vi "unmarshalling.vi"(7 "Type":variant, 8 "error in (no error)":errorcluster, 10 "String":string, 11 "Serializer in":refnum<class "Serializer.openg-ini.lvclass">) -> (0 "error out":errorcluster, 2 "Variant":variant, 3 "Serializer":refnum<class "Serializer.openg-ini.lvclass">)   [LabVIEW 2019, in "OpenSerializer.OpenG-ini.lvlib" / "Serializer.openg-ini.lvclass"]
uses:
  Serializer.openg-ini.lvclass
  Serializer.openg-ini.lvclass/Serializer.openg-ini.ctl
  <vilib>/Utility/config.llb/NI_LVConfig.lvlib
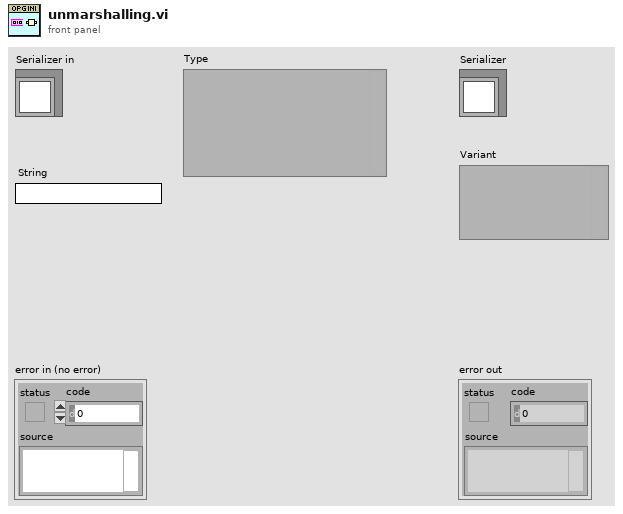
[diagram p1: front panel]
types:
  T1 = enum16{"open", "replace", "create", "open or create", "replace or create", "replace or create with confirmation"}
  T2 = typedef "NI_LVConfig.lvlib/Config Data RefNum.ctl" = refnum<k1>
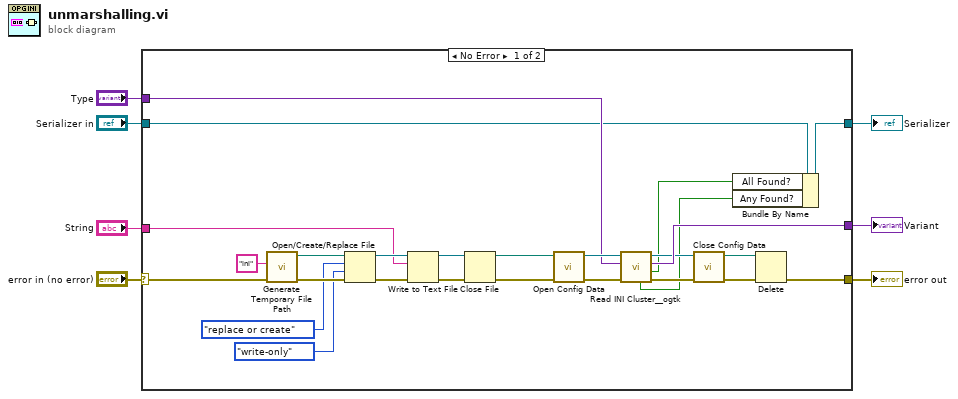
[diagram p0: block diagram]
diagram:
  n1 = case shown="No Error" "error in (no error)" {
    selector: "error in (no error)" -> [w32 w34]
    tunnel: "Serializer in" -> [w11 w35]
    tunnel: "String" -> [w25 _]
    tunnel: [w12 w35] -> w5
    tunnel: [w9 w34] -> w4
    tunnel: [w16 _] -> w3
    tunnel: "Type" -> [w17 _]
    frame No Error {
      n2 = call <vilib>:"Generate Temporary File Path.vi"("error in (no error)"=w32, "Temporary File Extension (tmp)"="ini") -> ("error out"=w30:errorcluster, "Unique Temporary File Path"=w31:path)  [unwired: 8 in]
      n3 = Open/Create/Replace File(file path (use dialog)=w31, error in=w30, operation (0:open)=T1."replace or create", access (0:read/write)=enum16{"read/write", "read-only", "write-only"}."write-only") -> (refnum out=w27:refnum<file>, error out=w26:errorcluster)  [unwired: 2 in, 1 out]
      n4 = Write to Text File(file (use dialog)=w27, text=w25, error in=w26) -> (refnum out=w23:refnum<file>, error out=w24:errorcluster)  [unwired: 1 in, 1 out]
      n5 = Close File(refnum=w23, error in=w24) -> (path=w21:path, error out=w22:errorcluster)
      n6 = call <vilib>:"Open Config Data.vi"("error in (no error)"=w22, "configuration file path"=w21) -> ("error out"=w20:errorcluster, "refnum"=w18:T2)  [unwired: 7 in, 1 out]
      n7 = call <userlib>:"Read INI Cluster__ogtk.vi"("error in (no error)"=w20, "INI Fomatted Cluster Type"=w17, "refnum"=w18) -> ("error out"=w19:errorcluster, "all found?"=w14:bool, "INI Fomatted Cluster"=w16:variant, "dup refnum"=w15:T2, "any found?"=w13:bool)  [unwired: 4 in]
      n8 = call <vilib>:"Close Config Data.vi"("error in (no error)"=w19, "refnum"=w15) -> ("error out"=w10:errorcluster, "file path"=w8:path)  [unwired: 8 in]
      n9 = Bundle By Name(cluster=w11, "All Found?"=w14, "Any Found?"=w13) -> (w12:refnum<class "Serializer.openg-ini.lvclass">)
      n10 = Delete(path (use dialog)=w8, error in=w10) -> (error out=w9:errorcluster)  [unwired: 3 in, 2 out]
    }
    frame Error {
    }
  }
  "error out" <- w4
  "Serializer" <- w5
  "Variant" <- w3
